vi "_StopSignal-GetSignalDefaultOrder.vi"(6 "LIBNAME":string, 8 "error in (no error)":errorcluster) -> (0 "error out":errorcluster, 2 "SignalInArray":string[](array[string]))   [LabVIEW 2017, in "StopSignal.lvlib"]
uses:
  StopSignal.lvlib
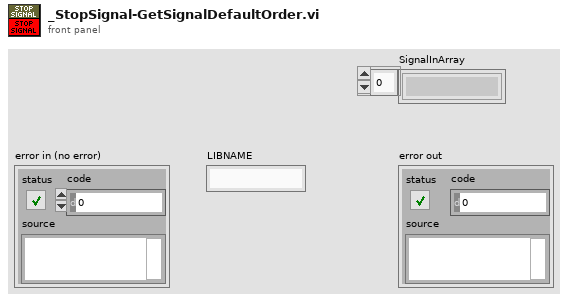
[diagram p1: front panel]
types:
  T1 = cluster{"ObjMap":variant, "CntMap":variant, "SignalInArray":string[]}
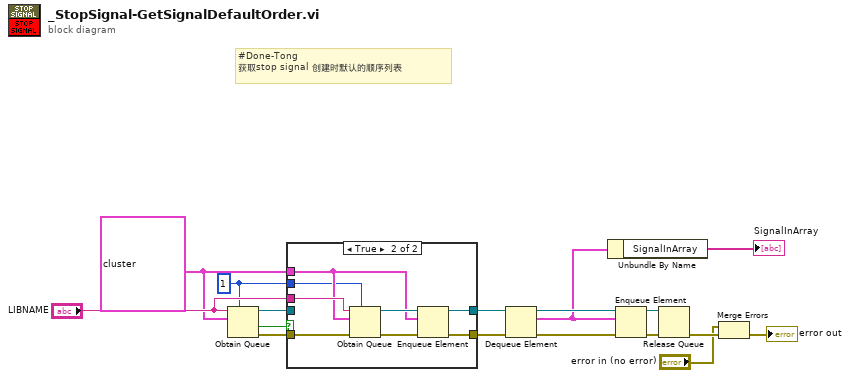
[diagram p0: block diagram]
diagram:
  w4 = T1 {"ObjMap"=variant, "CntMap"=variant, "SignalInArray"=[]}
  w5 = 1 ("max queue size (-1, unlimited)")
  # "#Done-Tong\n获取stop signal 创建时默认的顺序列表"
  n1 = Obtain Queue(max queue size (-1, unlimited)=w5, name (unnamed)="LIBNAME", element data type=w4) -> (queue out=w14:refnum<queue>, created new?=w16:bool, error out=w15:errorcluster)  [unwired: 2 in]
  n2 = case shown="True" w16 {
    tunnel: w15 -> [w18 w25]
    tunnel: w14 -> [w19 _]
    tunnel: w4 -> [_ w21]
    tunnel: [w18 w27] -> w13
    tunnel: [w19 w26] -> w12
    tunnel: "LIBNAME" -> [_ w22]
    tunnel: w5 -> [_ w20]
    frame False {
    }
    frame True {
      n3 = Obtain Queue(max queue size (-1, unlimited)=w20, name (unnamed)=w22, element data type=w21, error in (no error)=w25) -> (queue out=w23:refnum<queue>, error out=w24:errorcluster)  [unwired: 1 in, 1 out]
      n4 = Enqueue Element(queue=w23, element=w21, error in (no error)=w24) -> (queue out=w26:refnum<queue>, error out=w27:errorcluster)  [unwired: 1 in, 1 out]
    }
  }
  n5 = Dequeue Element(queue=w12, error in (no error)=w13) -> (queue out=w11:refnum<queue>, element=w2:T1, error out=w3:errorcluster)  [unwired: 1 in, 1 out]
  n6 = Unbundle By Name(w2) -> ("SignalInArray"=→"SignalInArray":string[])
  n7 = Enqueue Element(queue=w11, element=w2, error in (no error)=w3) -> (queue out=w10:refnum<queue>, error out=w9:errorcluster)  [unwired: 1 in, 1 out]
  n8 = Release Queue(queue=w10, error in (no error)=w9) -> (error out=w17:errorcluster)  [unwired: 1 in, 2 out]
  n9 = Merge Errors("error in (no error)", w17) -> (→"error out":errorcluster)
